vi "MAT Determine Data Type.vi"(0 "DBL":dbl[][](array[numeric]) format="%.2f", 1 "SGL":sgl[][](array[numeric]) format="%.2f", 2 "I32":i32[][](array[numeric]), 3 "I16":i16[][](array[numeric]), 4 "U16":u16[][](array[numeric]), 5 "U8":u8[][](array[numeric]), 6 "CDB":cdb[][](array[numeric]) format="%.2f", 7 "CSG":csg[][](array[numeric]) format="%.2f", 9 "STR":string[](array[string]), 13 "error in (no error)":errorcluster) -> (10 "Matrix Size":i32[](array[numeric]), 12 "Rep. Code":u32, 14 "Real/Complex (0-Real)":u32, 15 "error out":errorcluster, 17 "Representation":T1, 20 "DBL copy":dbl[][](array[numeric]) format="%.2f", 21 "SGL copy":sgl[][](array[numeric]) format="%.2f", 22 "I32 copy":i32[][](array[numeric]), 23 "I16 copy":i16[][](array[numeric]), 24 "U16 copy":u16[][](array[numeric]), 25 "U8 copy":u8[][](array[numeric]), 26 "CDB copy":cdb[][](array[numeric]) format="%.2f", 27 "CSG copy":csg[][](array[numeric]) format="%.2f")   [LabVIEW 2020, in "GOLPI library.lvlib"]
doc: "A subVI of Save to MAT. If more than one input contains a non-empty array, error is generated (error code 501)."
uses:
  GOLPI library.lvlib
  MAT Type Representation.ctl
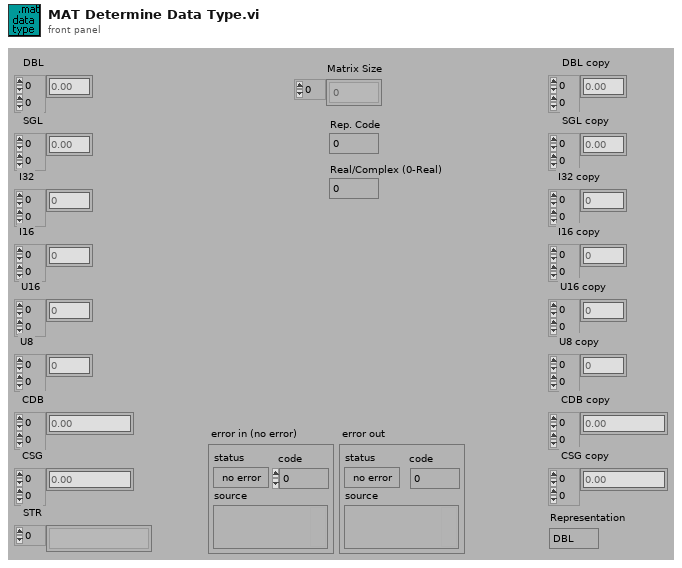
[diagram p1: front panel]
types:
  T1 = typedef "GOLPI library.lvlib/MAT Type Representation.ctl" = enum16{"DBL", "SGL", "I32", "I16", "U16", "U8", "CDB", "CSG", "STR"}
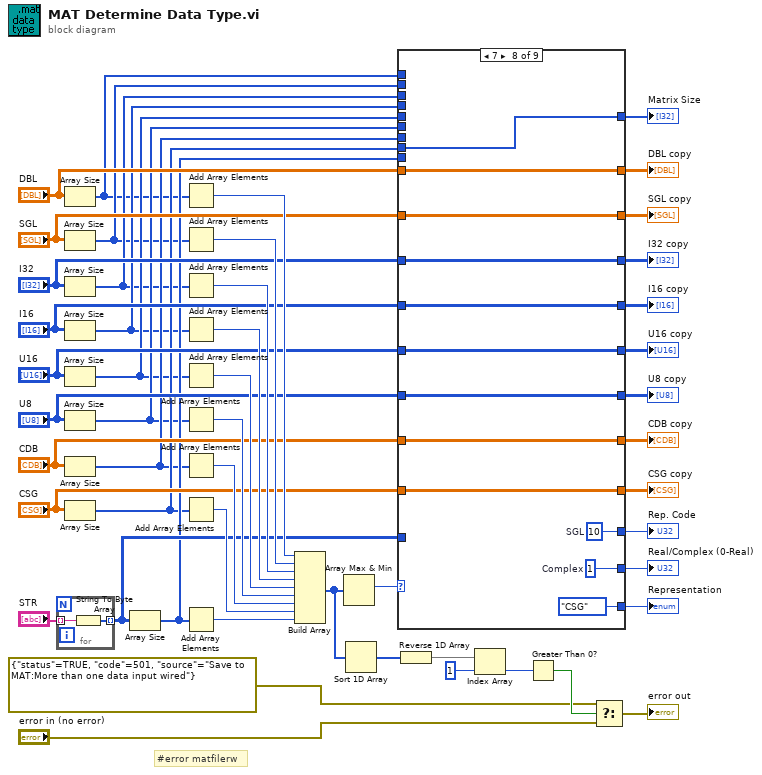
[diagram p0: block diagram]
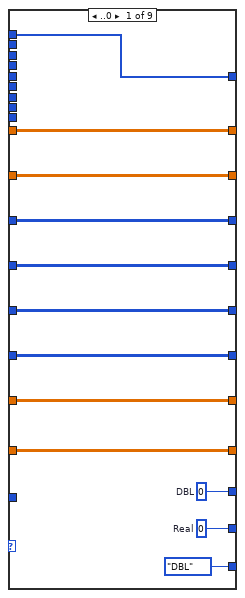
[diagram p2: hidden frame]
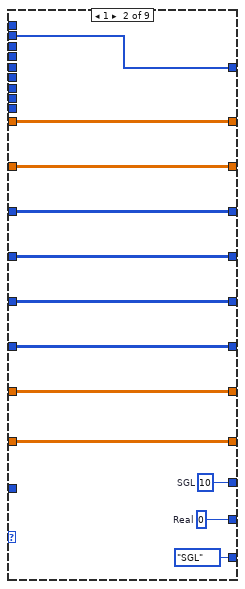
[diagram p3: hidden frame]
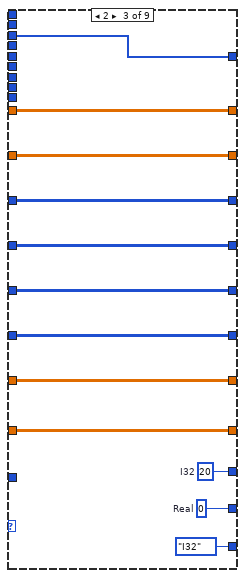
[diagram p4: hidden frame]
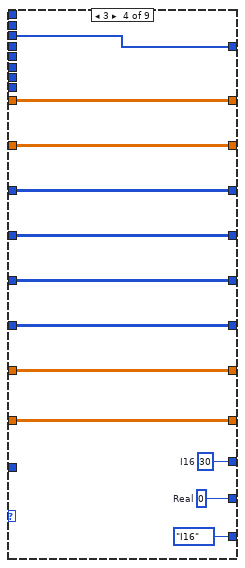
[diagram p5: hidden frame]
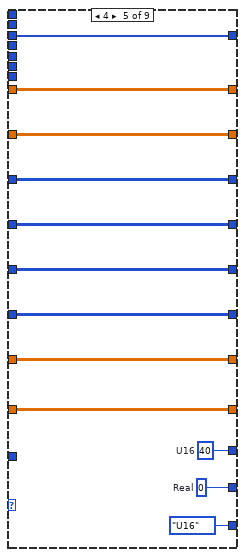
[diagram p6: hidden frame]
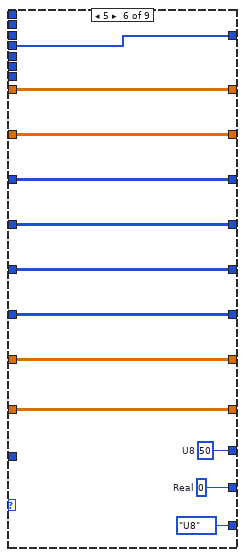
[diagram p7: hidden frame]
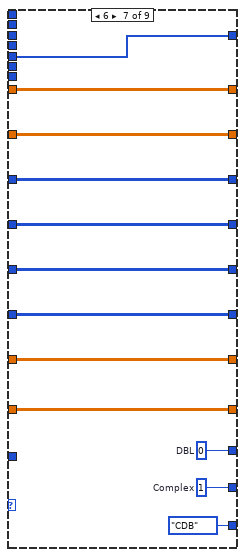
[diagram p8: hidden frame]
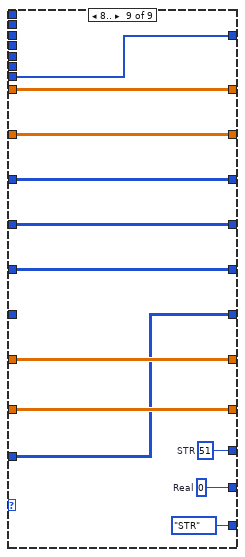
[diagram p9: hidden frame]
diagram:
  # "#error matfilerw"
  n1 = for {
    tunnel: "STR" -> [w52] mode=indexing
    tunnel: [w51] -> w24 mode=indexing
    n2 = String To Byte Array(string=w52) -> (unsigned byte array=w51:u8[])
  }
  n3 = Array Size(array="DBL") -> (size(s)=w13:i32[])
  n4 = Array Size(array="SGL") -> (size(s)=w14:i32[])
  n5 = Array Size(array="I32") -> (size(s)=w15:i32[])
  n6 = Array Size(array="I16") -> (size(s)=w16:i32[])
  n7 = Array Size(array="U16") -> (size(s)=w17:i32[])
  n8 = Array Size(array="U8") -> (size(s)=w18:i32[])
  n9 = Array Size(array="CDB") -> (size(s)=w19:i32[])
  n10 = Array Size(array="CSG") -> (size(s)=w20:i32[])
  n11 = Array Size(array=w24) -> (size(s)=w21:i32[])
  n12 = Add Array Elements(numeric array=w13) -> (sum=w49:i32)
  n13 = Add Array Elements(numeric array=w14) -> (sum=w48:i32)
  n14 = Add Array Elements(numeric array=w15) -> (sum=w47:i32)
  n15 = Add Array Elements(numeric array=w16) -> (sum=w46:i32)
  n16 = Add Array Elements(numeric array=w17) -> (sum=w45:i32)
  n17 = Add Array Elements(numeric array=w18) -> (sum=w44:i32)
  n18 = Add Array Elements(numeric array=w19) -> (sum=w43:i32)
  n19 = Add Array Elements(numeric array=w20) -> (sum=w42:i32)
  n20 = Add Array Elements(numeric array=w21) -> (sum=w41:i32)
  n21 = Build Array(w49, w48, w47, w46, w45, w44, w43, w42, w41) -> (w9:i32[])
  n22 = Array Max & Min(array=w9) -> (max index (indices)=w11:i32)  [unwired: 3 out]
  n23 = Sort 1D Array(array=w9) -> (sorted array=w7:i32[])
  n24 = case shown="7" w11 {
    tunnel: [w64 w76 w88 w100 w112 w124 w136 w148 w160] -> w23
    tunnel: [w63 w75 w87 w99 w111 w123 w135 w147 w159] -> w22
    tunnel: "DBL" -> [w53 w68 w81 w94 w107 w120 w133 w146 w158]
    tunnel: "SGL" -> [w62 w65 w80 w93 w106 w119 w132 w145 w157]
    tunnel: "I32" -> [w61 w74 w77 w92 w105 w118 w131 w144 w156]
    tunnel: "I16" -> [w60 w73 w86 w89 w104 w117 w130 w143 w155]
    tunnel: "U16" -> [w59 w72 w85 w98 w101 w116 w129 w142 w154]
    tunnel: "U8" -> [w58 w71 w84 w97 w110 w113 w128 w141 _]
    tunnel: "CDB" -> [w57 w70 w83 w96 w109 w122 w125 w140 w153]
    tunnel: "CSG" -> [w56 w69 w82 w95 w108 w121 w134 w137 w152]
    tunnel: [w53 w68 w81 w94 w107 w120 w133 w146 w158] -> w31
    tunnel: [w62 w65 w80 w93 w106 w119 w132 w145 w157] -> w30
    tunnel: [w61 w74 w77 w92 w105 w118 w131 w144 w156] -> w29
    tunnel: [w60 w73 w86 w89 w104 w117 w130 w143 w155] -> w28
    tunnel: [w58 w71 w84 w97 w110 w113 w128 w141 w149] -> w26
    tunnel: [w56 w69 w82 w95 w108 w121 w134 w137 w152] -> w32
    tunnel: [w59 w72 w85 w98 w101 w116 w129 w142 w154] -> w27
    tunnel: [w57 w70 w83 w96 w109 w122 w125 w140 w153] -> w25
    tunnel: w24 -> [_ _ _ _ _ _ _ _ w149]
    tunnel: w21 -> [_ _ _ _ _ _ _ _ w151]
    tunnel: w20 -> [_ _ _ _ _ _ _ w139 _]
    tunnel: w19 -> [_ _ _ _ _ _ w127 _ _]
    tunnel: w18 -> [_ _ _ _ _ w115 _ _ _]
    tunnel: w17 -> [_ _ _ _ w103 _ _ _ _]
    tunnel: w16 -> [_ _ _ w91 _ _ _ _ _]
    tunnel: w15 -> [_ _ w79 _ _ _ _ _ _]
    tunnel: w14 -> [_ w67 _ _ _ _ _ _ _]
    tunnel: w13 -> [w55 _ _ _ _ _ _ _ _]
    tunnel: [w55 w67 w79 w91 w103 w115 w127 w139 w151] -> w12
    tunnel: [MAT_Type_Representation."DBL" ("Representation") MAT_Type_Representation."SGL" ("Representation") MAT_Type_Representation."I32" ("Representation") MAT_Type_Representation."I16" ("Representation") MAT_Type_Representation."U16" ("Representation") MAT_Type_Representation."U8" ("Representation") MAT_Type_Representation."CDB" ("Representation") MAT_Type_Representation."CSG" ("Representation") MAT_Type_Representation."STR" ("Representation")] -> w10
    frame ..0 {
      w63 = u32 0  # Real
      w64 = u32 0  # DBL
    }
    frame 1 {
      w75 = u32 0  # Real
      w76 = u32 10  # SGL
    }
    frame 2 {
      w87 = u32 0  # Real
      w88 = u32 20  # I32
    }
    frame 3 {
      w99 = u32 0  # Real
      w100 = u32 30  # I16
    }
    frame 4 {
      w111 = u32 0  # Real
      w112 = u32 40  # U16
    }
    frame 5 {
      w123 = u32 0  # Real
      w124 = u32 50  # U8
    }
    frame 6 {
      w135 = u32 1  # Complex
      w136 = u32 0  # DBL
    }
    frame 7 {
      w147 = u32 1  # Complex
      w148 = u32 10  # SGL
    }
    frame 8.. {
      w159 = u32 0  # Real
      w160 = u32 51  # STR
    }
  }
  "DBL copy" <- w31
  "SGL copy" <- w30
  "CSG copy" <- w32
  "I32 copy" <- w29
  "I16 copy" <- w28
  "U16 copy" <- w27
  "U8 copy" <- w26
  "CDB copy" <- w25
  "Matrix Size" <- w12
  "Rep. Code" <- w23
  "Real/Complex (0-Real)" <- w22
  "Representation" <- w10
  n25 = Reverse 1D Array(array=w7) -> (reversed array=w6:i32[])
  n26 = Index Array(array=w6, index=1) -> (element=w5:i32)
  n27 = Greater Than 0?(x=w5) -> (x > 0?=w4:bool)
  n28 = Select(t=errorcluster {"status"=TRUE, "code"=501, "source"="Save to MAT:More than one data input wired"} ("error in (no error)"), s=w4, f="error in (no error)") -> (s? t:f=→"error out":errorcluster)
